vi "Configure-cameras.vi"(8 "error in":errorcluster, 11 "Data ref. in":refnum<data-value>) -> (0 "error IO":errorcluster, 3 "Data ref.":refnum<data-value>, 4 "Initialized?":bool, 5 "Succes?":bool)   [LabVIEW 2013, in "CameraVision.lvlib" / "CV-Main.lvclass"]
doc: "This function initializes the framegrabber hardware (the hardware between the camera and the pc).\nThe necessary memory resources are calculated and allocated.\nThe configuration settings for the framegrabber are loaded from the user selected configuration file and updated with the parameter values from the GUI controls.\n\nSeparate error messages are displayed when either the user selected framegrabber configuration file is corrupted or when the communication to the framegrabber fails."
uses:
  CV-Main.lvclass
  CV-Main.lvclass/CV-Main.ctl
  UI/Module-states.ctl
  Read Acquis params.vi
  Read Config params.vi
  Read Correct params.vi
  Acquisition/CV-Acquisition.lvclass
  Configuration/CV-Configuration.lvclass
  Correction/CV-Correction.lvclass
  UI/CV-UI.lvclass
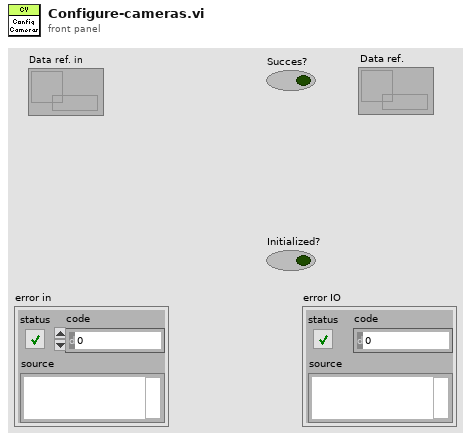
[diagram p1: front panel]
types:
  T1 = typedef "CameraVision.lvlib/CV-UI.lvclass/Module-states.ctl" = enum16{"Inactive", "Active", "Data-loss", "Error", "Simulation", "Synchronizing", "Initialized", "Released"}
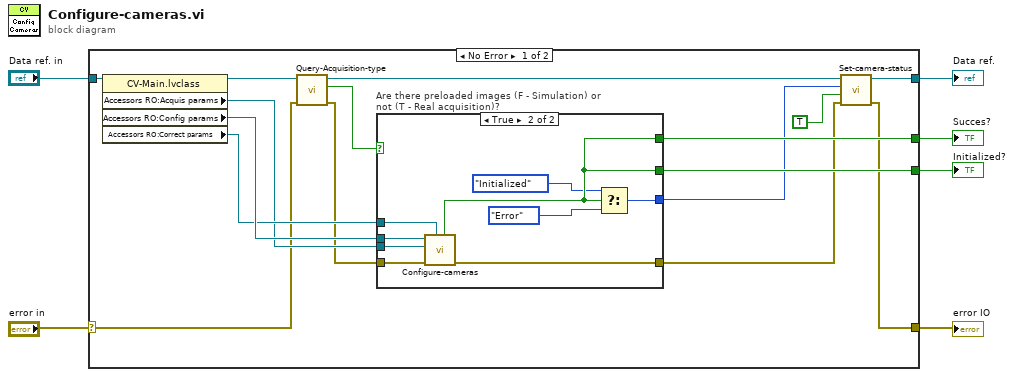
[diagram p0: block diagram]
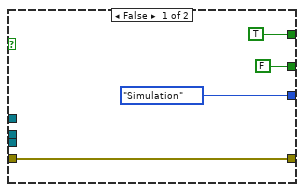
[diagram p2: hidden frame]
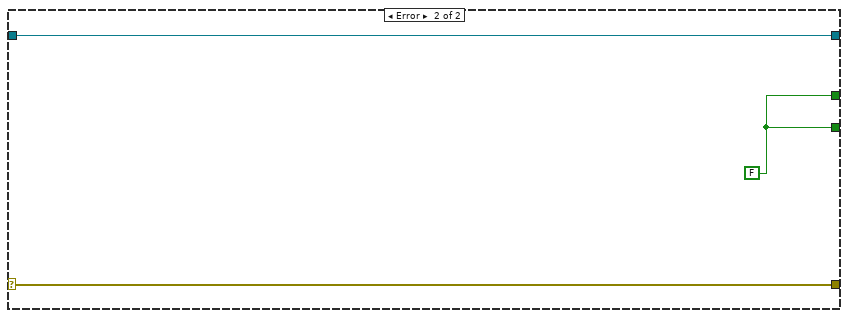
[diagram p3: hidden frame]
diagram:
  n1 = case shown="No Error" "error in" {
    selector: "error in" -> [w17 w38]
    tunnel: [w21 w37] -> w6
    tunnel: [w7 w38] -> w5
    tunnel: [w22 w37] -> w3
    tunnel: "Data ref. in" -> [w14 w36]
    tunnel: [w11 w36] -> w1
    frame No Error {
      n2 = property class="CV-Main.lvclass"(reference=w14) -> (reference out=w13:refnum<data-value>, "Accessors RO:Acquis params"=w18:refnum<data-value>, "Accessors RO:Config params"=w20:refnum<data-value>, "Accessors RO:Correct params"=w19:refnum<data-value>)  [unwired: 1 in, 1 out]
      n3 = call "Query-Acquisition-type.vi"("error in"=w17, "Data ref. in"=w13) -> ("error IO"=w16:errorcluster, "Hardware acquisiton?"=w15:bool, "Data ref."=w12:refnum<data-value>)  [unwired: 7 in]
      n4 = case "Are there preloaded images (F - Simulation) or not (T - Real acquisition)?" shown="True" w15 {
        tunnel: [FALSE w30] -> w22
        tunnel: [w25 w35] -> w10
        tunnel: w16 -> [w25 w34]
        tunnel: [TRUE ("Succes?") w30] -> w21
        tunnel: w20 -> [_ w27]
        tunnel: w19 -> [_ w33]
        tunnel: w18 -> [_ w32]
        tunnel: [Module-states."Simulation" ("Camera status") w31] -> w9
        frame False {
        }
        frame True {
          n5 = call "Configure-cameras.vi"("Correct. params. ref."=w33, "error in"=w34, "Acquis. params. ref."=w32, "Config. params. ref in."=w27) -> ("error IO"=w35:errorcluster, "Succes?"=w30:bool)  [unwired: 5 in, 1 out]
          n6 = Select(t=Module-states."Initialized" ("Camera status"), s=w30, f=Module-states."Error" ("Camera status")) -> (s? t:f=w31:T1)
        }
      }
      n7 = call "Set-camera-status.vi"("error in"=w10, "Reset errors?"=TRUE, "Cam. status in"=w9, "Data ref. in"=w12) -> ("error IO"=w7:errorcluster, "Data ref."=w11:refnum<data-value>)  [unwired: 5 in, 1 out]
    }
    frame Error {
      w37 = FALSE
    }
  }
  "Succes?" <- w6
  "error IO" <- w5
  "Initialized?" <- w3
  "Data ref." <- w1
